vi "myRIO_Brig_Host_comm_webdav_uploadFile__settings.vi"(8 "input_error":errorcluster, 9 "input_filePath_local":path, 10 "dataName":string="dataExp", 11 "input_hSession":T1) -> (0 "output_error":errorcluster, 2 "output_Iexist":bool, 3 "output_hSession":T1)   [LabVIEW 2014]
uses:
  <vilib>/WebDAVClient/Advanced/SessionHandle.ctl
  <vilib>/WebDAVClient/Advanced/Put File.vi
  <vilib>/WebDAVClient/NI_WebDAV.lvlib
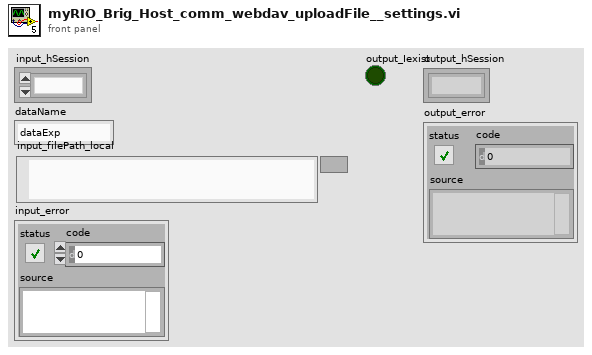
[diagram p1: front panel]
types:
  T1 = typedef "NI_WebDAV.lvlib/SessionHandle.ctl" = refnum<k1>
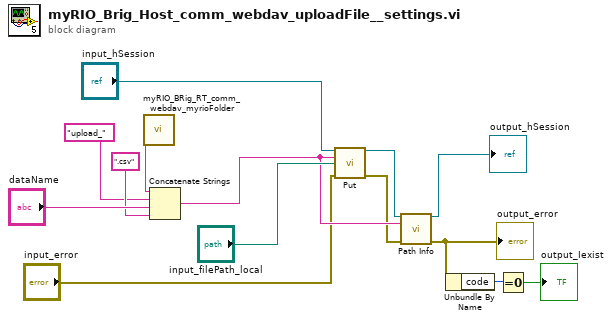
[diagram p0: block diagram]
diagram:
  n1 = call "myRIO_BRig_RT_comm_webdav_myrioFolder.vi"() -> ("output_myrioFolder"=w11:string)  [unwired: 11 in]
  n2 = Concatenate Strings(w11, "upload_" ("string"), "dataName", ".csv" ("string")) -> (w7:string)
  n3 = call-poly <vilib>:"Put.vi"("session handle"="input_hSession", "relative uri"=w7, "local file path"="input_filePath_local", "error in (no error)"="input_error") -> ("session handle out"=w8:T1, "error out"=w6:errorcluster)  [unwired: 9 in, 1 out]
  n4 = call <vilib>:"Path Info.vi"("session handle"=w8, "relative uri"=w7, "error in (no error)"=w6) -> ("session handle out"=→"output_hSession":T1, "error out"=w4:errorcluster)  [unwired: 9 in, 2 out]
  "output_error" <- w4
  n5 = Unbundle By Name(w4) -> ("code"=w3:i32)
  n6 = Equal To 0?(x=w3) -> (x = 0?=→"output_Iexist":bool)
